vi "ActBegin.vi"(8 "error in (no error)":errorcluster) -> (0 "error out":errorcluster)   [LabVIEW 2023]
doc: "Creates any refrences and begins any functions for the action system. (Probably Useless)\ninput: \n -- error in -- cluster\n\noutput:\n -- error out -- cluster"
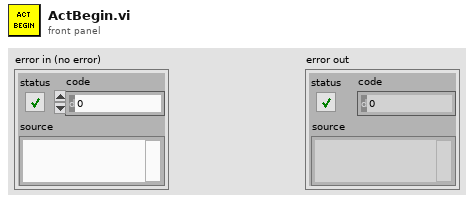
[diagram p1: front panel]
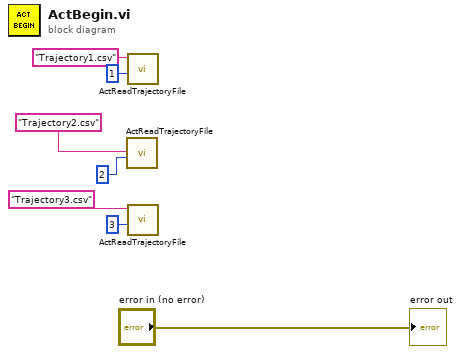
[diagram p0: block diagram]
diagram:
  n1 = call "ActReadTrajectoryFile.vi"("Index 1,2,3,4"=2, "FileName"="Trajectory2.csv") -> ()  [unwired: 10 in]
  n2 = call "ActReadTrajectoryFile.vi"("Index 1,2,3,4"=1, "FileName"="Trajectory1.csv") -> ()  [unwired: 10 in]
  n3 = call "ActReadTrajectoryFile.vi"("Index 1,2,3,4"=3, "FileName"="Trajectory3.csv") -> ()  [unwired: 10 in]
  "error out" <- "error in (no error)"
